vi "WebSocket Handshake.vi"(8 "error in (no error)":errorcluster, 11 "Function in":refnum<class "Function.lvclass">) -> (0 "error out":errorcluster, 3 "Function out":refnum<class "Function.lvclass">)   [LabVIEW 2016, in "Function Actor.lvlib" / "Function.lvclass"]
uses:
  <userlib>/Common Components/Function Actor/Function.lvclass
  C:/Program Files (x86)/National Instruments/LabVIEW 2016/vi.lib/ActorFramework/Actor/Actor.lvclass
  <userlib>/Common Components/Function Messages/WebSocket Handshake Msg/WebSocket Handshake Msg.lvclass
  C:/Program Files (x86)/National Instruments/LabVIEW 2016/vi.lib/ActorFramework/Message/Message.lvclass
  <vilib>/ActorFramework/Actor/Actor.lvclass/Actor.ctl
  <vilib>/ActorFramework/Message Enqueuer/Message Enqueuer.lvclass/Message Enqueuer.ctl
  <userlib>/Common Components/Function Actor/Function.lvclass/Function.ctl
  <vilib>/ActorFramework/Message Enqueuer/Init from Existing Queue.vi
  <vilib>/ActorFramework/Message Enqueuer/Message Enqueuer.lvclass
  <vilib>/MediaMongrels Ltd/WebSockets/WebSockets/WebSockets.lvlib
  <vilib>/ActorFramework/Actor/Actor.lvclass
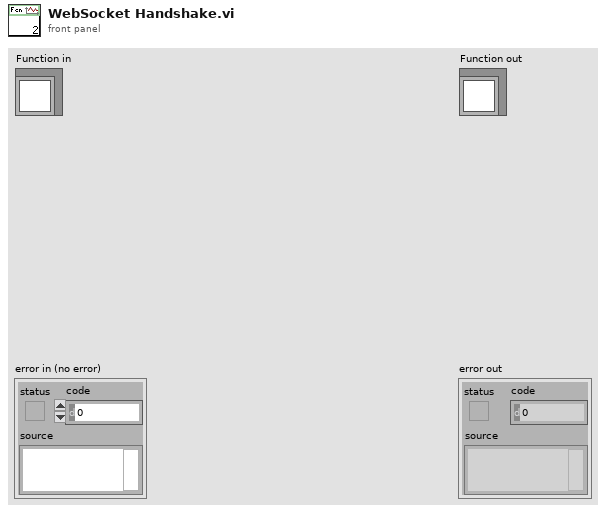
[diagram p1: front panel]
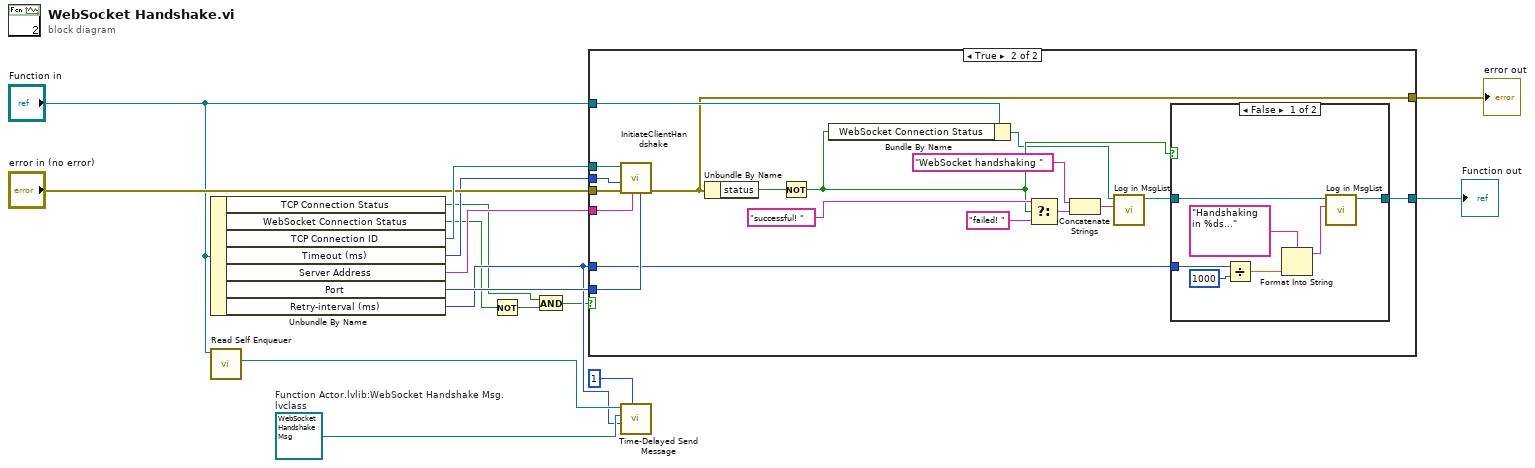
[diagram p0: block diagram]
diagram:
  w7 = refnum<class "WebSocket Handshake Msg.lvclass"> refnum  # Function Actor.lvlib:WebSocket Handshake Msg.lvclass
  n1 = Unbundle By Name("Function in") -> ("TCP Connection Status"=w4:bool, "WebSocket Connection Status"=w3:bool, "TCP Connection ID"=w16:refnum<k5>, "Timeout (ms)"=w14:i32, "Server Address"=w13:string, "Port"=w12:u16, "Retry-interval (ms)"=w5:i32)
  n2 = call <vilib>:"Read Self Enqueuer.vi"("Actor"="Function in") -> ("Self Enqueuer"=w9:refnum<class "Message Enqueuer.lvclass">)  [unwired: 10 in]
  n3 = Not(x=w3) -> (.not. x?=w2:bool)
  n4 = And(x=w4, y=w2) -> (x .and. y?=w1:bool)
  n5 = case shown="True" w1 {
    tunnel: "Function in" -> [w17 w36]
    tunnel: w16 -> [_ w35]
    tunnel: "error in (no error)" -> [w18 w34]
    tunnel: w14 -> [_ w33]
    tunnel: w13 -> [_ w32]
    tunnel: w12 -> [_ w31]
    tunnel: [w18 w30] -> w11
    tunnel: [w17 w20] -> w10
    tunnel: w5 -> [_ w19]
    frame False {
    }
    frame True {
      n6 = call <vilib>:"InitiateClientHandshake.vi"("remote port or service name"=w31, "address"=w32, "error in (no error)"=w34, "timeout ms (5000)"=w33, "WebSocket Connection in"=w35) -> ("error out"=w30:errorcluster)  [unwired: 4 in, 2 out]
      n7 = Unbundle By Name(w30) -> ("status"=w29:bool)
      n8 = Not(x=w29) -> (.not. x?=w22:bool)
      n9 = Bundle By Name(cluster=w36, "WebSocket Connection Status"=w22) -> (w21:refnum<class "Function.lvclass">)
      n10 = Select(t="successful! ", s=w22, f="failed! ") -> (s? t:f=w25:string)
      n11 = Concatenate Strings("WebSocket handshaking ", w25) -> (w24:string)
      n12 = call-dynamic "Log in MsgList.vi"("Msg"=w24, "Function in"=w21) -> ("Function out"=w23:refnum<class "Function.lvclass">)  [unwired: 8 in, 1 out]
      n13 = case shown="False" w22 {
        tunnel: w23 -> [w42 w44]
        tunnel: [w43 w44] -> w20
        tunnel: w19 -> [w38 _]
        frame False {
          n14 = Divide(x=w38, y=1000) -> (x/y=w39:dbl)
          n15 = Format Into String(format string="Handshaking in %ds..." ("Msg"), w39) -> (resulting string=w40:string)  [unwired: 2 in, 1 out]
          n16 = call-dynamic "Log in MsgList.vi"("Msg"=w40, "Function in"=w42) -> ("Function out"=w43:refnum<class "Function.lvclass">)  [unwired: 8 in, 1 out]
        }
        frame True {
        }
      }
    }
  }
  "error out" <- w11
  "Function out" <- w10
  n17 = call <vilib>:"Time-Delayed Send Message.vi"("# Copies (0 = infinite repeat)"=u32 1, "Milliseconds To Wait"=w5, "Message"=w7, "Message Enqueuer"=w9) -> ()  [unwired: 6 in, 2 out]
